vi "get default reporter.vi"(8 "error in":errorcluster, 11 "dispatcher":refnum<data-value>) -> (0 "error out":errorcluster, 2 "default result reporter":refnum<class "results reporter.lvclass">, 3 "dispatcher out":refnum<data-value>)   [LabVIEW 2013, in "thread pool.lvclass"]
uses:
  thread pool.lvclass
  results reporter/results reporter.lvclass
  thread pool.lvclass/thread pool.ctl
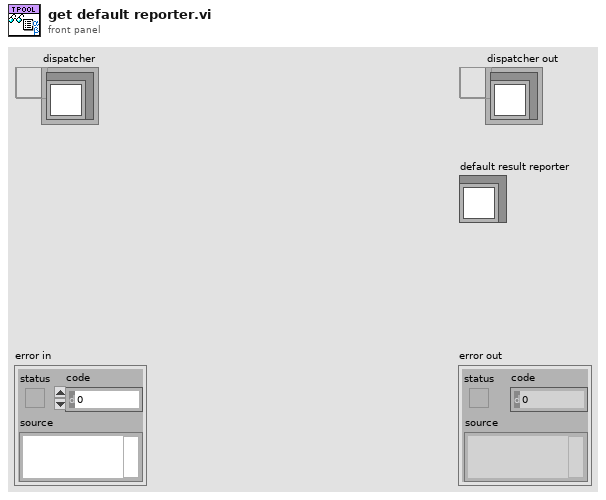
[diagram p1: front panel]
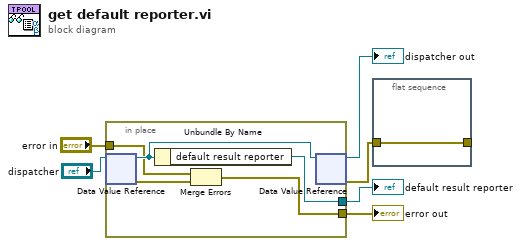
[diagram p0: block diagram]
diagram:
  n1 = in-place {
    in-place-border: [w10] -> w3
    in-place-border: "error in" -> [w8]
    in-place-border: [w7] -> w1
    n2 = in-place-dvr #1("dispatcher") -> (w11:refnum<class "thread pool.lvclass">, w9:errorcluster)
    n3 = Unbundle By Name(w11) -> ("default result reporter"=w7:refnum<class "results reporter.lvclass">)
    n4 = Merge Errors(w8, w9) -> (w10:errorcluster)
    n5 = in-place-dvr #1(w11) -> (→"dispatcher out":refnum<data-value>, w6:errorcluster)
  }
  "error out" <- w3
  "default result reporter" <- w1
  n6 = flat-sequence {
    tunnel: [w12] -> _
    tunnel: w6 -> [w12]
    frame #0 {
    }
  }
